vi "Improved F to C.vi"() -> ()   [LabVIEW 2021]
panel:
  in  "Boolean":bool
  out "Thermometer (C) 2":dbl(slide) scale=0.0..100.0
  in  "Thermometer (F) 2":dbl(slide) scale=0.0..100.0
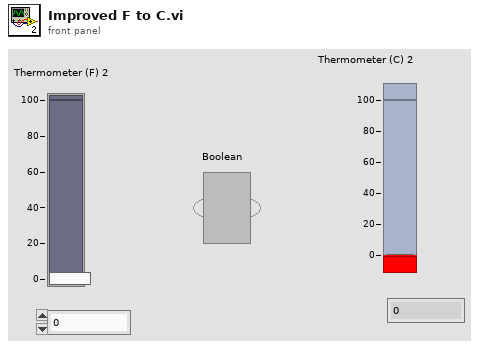
[diagram p1: front panel]
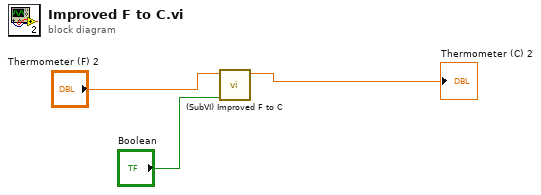
[diagram p0: block diagram]
diagram:
  n1 = call "(SubVI) Improved F to C.vi"("Boolean"="Boolean", "Thermometer (F) in"="Thermometer (F) 2") -> ("Numeric"=→"Thermometer (C) 2":dbl)  [unwired: 9 in]
